vi "Calc_Allan-Variance.VI"(1 "tau":i32, 2 "Input Array":dbl[](array[numeric]) format="%.2f") -> (0 "Allan-variance (tau)":dbl format="%.2f")   [LabVIEW 2021]
uses:
  <vilib>/Analysis/baseanly.llb/Mean (DBL).vi
  <vilib>/Analysis/NI_AALBase.lvlib
panel:
  out "[y_mean(k+1) - y_mean(k)]**2":dbl[](array[numeric]) format="%.3f"
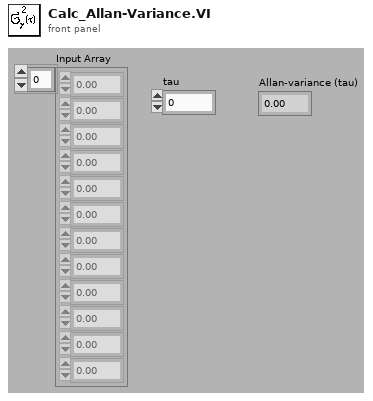
[diagram p1: front panel]
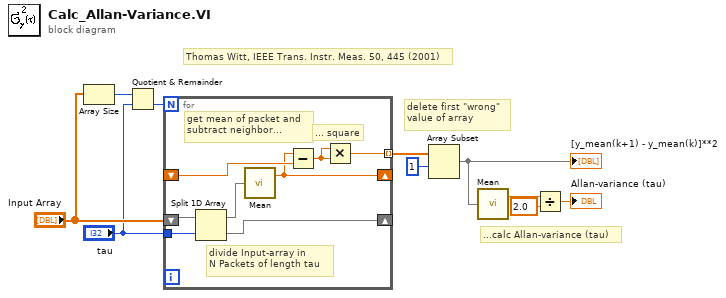
[diagram p0: block diagram]
diagram:
  # "Thomas Witt, IEEE Trans. Instr. Meas. 50, 445 (2001)"
  # "delete first \"wrong\"\nvalue of array"
  # "...calc Allan-variance (tau)"
  n1 = Array Size(array="Input Array") -> (size(s)=w10:i32)
  n2 = Quotient & Remainder(x=w10, y="tau") -> (floor(x/y)=w7:i32)  [unwired: 1 out]
  n3 = for {
    N: w7 -> [_]
    shift-right: [w17] -> _
    shift-left: "Input Array" -> [w18]
    tunnel: "tau" -> [w11]
    shift-right: [w14] -> _
    shift-left: _ -> [w15]
    tunnel: [w12] -> w3 mode=indexing
    # "... square"
    # "get mean of packet and\nsubtract neighbor..."
    # "divide Input-array in\nN Packets of length tau"
    n4 = Split 1D Array(array=w18, index=w11) -> (first subarray=w16:dbl[], second subarray=w17:dbl[])
    n5 = call-poly <vilib>:"Mean.vi"("X"=w16) -> ("mean"=w14:dbl)  [unwired: 1 out]
    n6 = Subtract(x=w14, y=w15) -> (x-y=w13:dbl)
    n7 = Multiply(x=w13, y=w13) -> (x*y=w12:dbl)
  }
  n8 = Array Subset(array=w3, index=1 ("mean")) -> (w1:dbl[])  [unwired: 1 in]
  "[y_mean(k+1) - y_mean(k)]**2" <- w1
  n9 = call-poly <vilib>:"Mean.vi"("X"=w1) -> ("mean"=w6:dbl)  [unwired: 1 out]
  n10 = Divide(x=w6, y=2.0) -> (x/y=→"Allan-variance (tau)":dbl)
